vi "Sequence test.vi"() -> ()   [LabVIEW 2020, in "Toggle 6.lvclass"]
uses:
  Toggle 6.lvclass
  WS1041/WS1041.lvclass
  Controls/Change setting mode enum.ctl
  XML Handler/XML Handler.lvclass
  XML Handler/Controls/Result Cluster.ctl
  PIC-device/PIC-Device.lvclass
  Measurements/Measurement.lvclass
panel:
  out "Parameters Out":cluster{"Name":string, "Value":string}[](array[cluster])
  out "Changes":cluster{"Name":string, "Value":string}[](array[cluster])
  in  "Exit":bool
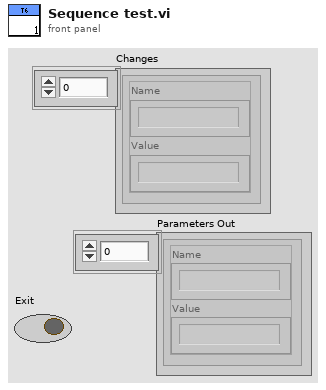
[diagram p1: front panel]
types:
  T1 = cluster{"Temperature [degC]":dbl, "Soak time [s]":dbl, "PSUs":cluster{"PSU alias":string, "Source":enum32{"Voltage", "Current"}, "Drive (V/A)":dbl}[]}
  T2 = typedef "PIC-Device.lvclass/Change setting mode enum.ctl" = enum16{"Init", "Next", "Reset"}
  T3 = typedef "XML Handler.lvclass/Result Cluster.ctl" = cluster{"Name":string, "Value":string}
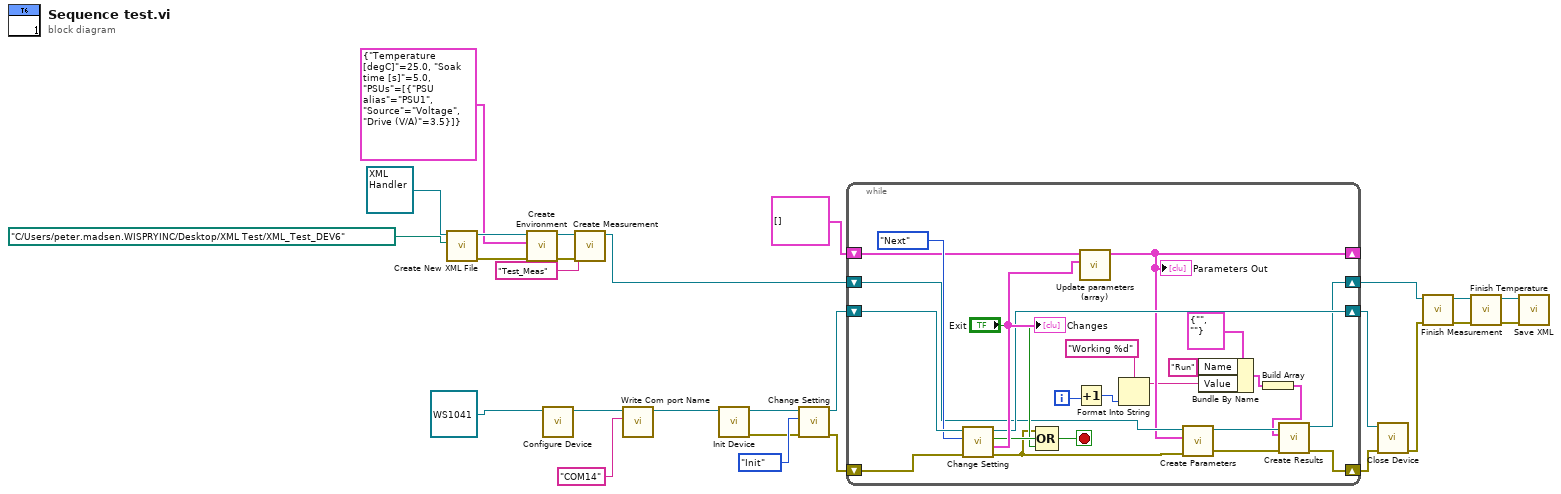
[diagram p0: block diagram]
diagram:
  n1 = call "Create New XML File.vi"("Output File Folder"=path "C:/Users/peter.madsen.WISPRYINC/Desktop/XML Test/XML_Test_DEV6", "XML Handler in"=refnum<class "XML Handler.lvclass"> refnum ("XML Handler.lvclass")) -> ("error out"=w13:errorcluster, "XML Handler out"=w12:refnum<class "XML Handler.lvclass">)  [unwired: 8 in]
  n2 = call "Create Environment.vi"("error in (no error)"=w13, "Environmental info"=T1 {"Temperature [degC]"=25.0, "Soak time [s]"=5.0, "PSUs"=[{"PSU alias"="PSU1", "Source"=enum."Voltage", "Drive (V/A)"=3.5}]}, "XML Handler in"=w12) -> ("error out"=w11:errorcluster, "XML Handler out"=w10:refnum<class "XML Handler.lvclass">)  [unwired: 7 in]
  n3 = call-dynamic "Configure Device.vi"("WS1041 in"=refnum<class "WS1041.lvclass"> refnum ("WS1041.lvclass")) -> ("WS1041 out"=w19:refnum<class "WS1041.lvclass">)  [unwired: 9 in, 1 out]
  n4 = call "Create Measurement.vi"("error in (no error)"=w11, "Measurement Name"="Test_Meas", "XML Handler in"=w10) -> ("XML Handler out"=w8:refnum<class "XML Handler.lvclass">)  [unwired: 7 in, 1 out]
  n5 = call-dynamic "Write Com port Name.vi"("Com port Name"="COM14", "Device in"=w19) -> ("Device out"=w18:refnum<class "WS1041.lvclass">)  [unwired: 9 in]
  n6 = call-dynamic "Init Device.vi"("Toggle 6 in"=w18) -> ("error out"=w24:errorcluster, "Toggle 6 out"=w26:refnum<class "WS1041.lvclass">)  [unwired: 9 in]
  n7 = call-dynamic "Change Setting.vi"("error in (no error)"=w24, "Change setting mode"=Change_setting_mode_enum."Init", "Toggle 6 in"=w26) -> ("error out"=w22:errorcluster, "Toggle 6 out"=w23:refnum<class "WS1041.lvclass">)  [unwired: 5 in, 2 out]
  n8 = while {
    shift-right: [w39] -> w21
    shift-left: w22 -> [w51]
    shift-right: [w48] -> w20
    shift-left: w23 -> [w50]
    shift-right: [w40] -> _
    shift-left: cluster{"Name":string, "Value":string}[] [] ("Parameters Out") -> [w43]
    shift-right: [w36] -> w7
    shift-left: w8 -> [w41]
    i -> [w32]
    stop <- w45 stop-if-true
    n9 = call-dynamic "Change Setting.vi"("error in (no error)"=w51, "Change setting mode"=Change_setting_mode_enum."Next", "Toggle 6 in"=w50) -> ("error out"=w42:errorcluster, "Changes"=w49:cluster{"Name":string, "Value":string}[], "Last setting"=w47:bool, "Toggle 6 out"=w48:refnum<class "WS1041.lvclass">)  [unwired: 5 in]
    "Changes" <- w49
    n10 = Compound Arithmetic op=OR(w42, w47, "Exit") -> (w45:bool)
    n11 = Increment(x=w32) -> (x+1=w31:i32)
    n12 = call "Update parameters (array).vi"("New Parameters"=w49, "Parameters"=w43) -> ("Parameters Out"=w40:cluster{"Name":string, "Value":string}[])  [unwired: 9 in]
    "Parameters Out" <- w40
    n13 = Format Into String(format string="Working %d" ("Value"), w31) -> (resulting string=w30:string)  [unwired: 2 in, 1 out]
    n14 = call "Create Parameters.vi"("error in (no error)"=w42, "Parameters"=w40, "XML Handler in"=w41) -> ("error out"=w38:errorcluster, "XML Handler out"=w37:refnum<class "XML Handler.lvclass">)  [unwired: 7 in]
    n15 = Bundle By Name(cluster=T3 {"Name"="", "Value"=""} ("Result Cluster"), "Name"="Run", "Value"=w30) -> (w29:T3)
    n16 = Build Array(w29) -> (w28:T3[])
    n17 = call "Create Results.vi"("error in (no error)"=w38, "Results"=w28, "XML Handler in"=w37) -> ("error out"=w39:errorcluster, "XML Handler out"=w36:refnum<class "XML Handler.lvclass">)  [unwired: 7 in]
  }
  n18 = call-dynamic "Close Device.vi"("error in (no error)"=w21, "Device in"=w20) -> ("error out"=w4:errorcluster)  [unwired: 8 in, 1 out]
  n19 = call-dynamic "Finish Measurement.vi"("error in (no error)"=w4, "XML Handler in"=w7) -> ("error out"=w5:errorcluster, "XML Handler out"=w6:refnum<class "XML Handler.lvclass">)  [unwired: 8 in]
  n20 = call "Finish Temperature.vi"("error in (no error)"=w5, "XML Handler in"=w6) -> ("error out"=w3:errorcluster, "XML Handler out"=w2:refnum<class "XML Handler.lvclass">)  [unwired: 8 in]
  n21 = call "Save XML.vi"("error in (no error)"=w3, "XML Handler in"=w2) -> ()  [unwired: 8 in, 2 out]
